vi "MFLI_Messgerät.vi"(1 "refnum":refnum<file>, 2 "Numerisch":i8 min=0 max=2 step=1) -> ()   [LabVIEW 2019]
uses:
  Global/Global Variables/Data_Display_global.vi
  Instrument_Setup.vi
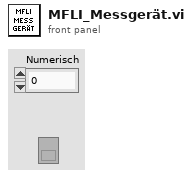
[diagram p1: front panel]
types:
  T1 = typedef "MFLIMonitor-Settings-Cluster.ctl" = cluster{"Adress":string, "Osc 0 Freq":dbl, "Osc 1 Freq":dbl, "Osc 2 Freq":dbl, "Osc 3 Freq":dbl, "Demod 0 Osc":i8, "Demod 0 Harm":i16, "Demod 0 Phase":dbl, "Demod 1 Osc":i8, "Demod 2 Osc":i8, "Demod 3 Osc":i8, "Demod 1 Harm":i16, "Demod 2 Harm":i16, "Demod 3 Harm":i16, "Demod 1 Phase":dbl, "Demod 2 Phase":dbl, "Demod 3 Phase":dbl, "Input Demod 0":string, "Input Demod 1":string, "Input Demod 2":string, "Input Demod 3":string, "Demod 0 Order":i8, "Demod 0 TC":dbl, "Demod 0 Sinc":bool, "Demod 1 Order":i8, "Demod 2 Order":i8, "Demod 3 Order":i8, "Demod 1 TC":dbl, "Demod 2 TC":dbl, "Demod 3 TC":dbl, "Demod 1 Sinc":bool, "Demod 2 Sinc":bool, "Demod 3 Sinc":bool, "Demod 0 Enable":bool, "Demod 0 Data Rate":dbl, "Demod 1 Enable":bool, "Demod 2 Enable":bool, "Demod 3 Enable":bool, "Demod 1 Data Rate":dbl, "Demod 2 Data Rate":dbl, "Demod 3 Data Rate":dbl, "Ampl 0":dbl, "Ampl 0 Enable":bool, "Ampl 1":dbl, "Ampl 2":dbl, "Ampl 3":dbl, "Ampl 1 Enable":bool, "Ampl 2 Enable":bool, "Ampl 3 Enable":bool, "On":bool, "50 Ohm":bool, "Range (V)":dbl, "Add":bool, "Diff":bool, "Auto-Range":bool, "Offset (V)":dbl, "Aux Out 0 Select":string, "Aux Out 0 Demod Num":dbl, "Aux Out 0 Pre Offset":dbl, "Aux Out 0 Scale":dbl, "Aux Out 0 Offset":dbl, "Aux Out 1 Select":string, "Aux Out 2 Select":string, "Aux Out 3 Select":string, "Aux Out 1 Pre Offset":dbl, "Aux Out 2 Pre Offset":dbl, "Aux Out 3 Pre Offset":dbl, "Aux Out 1 Scale":dbl, "Aux Out 2 Scale":dbl, "Aux Out 3 Scale":dbl, "Aux Out 1 Offset":dbl, "Aux Out 2 Offset":dbl, "Aux Out 3 Offset":dbl, "Aux Out 1 Demod Num":dbl, "Aux Out 2 Demod Num ":dbl, "Aux Out 3 Demod Num":dbl, "Output Range (V)":dbl}
  T2 = typedef "MFLIMonitor_Cluster.ctl" = cluster{"Demod 0":dbl[][], " Demod 1":dbl[][], "Demod 0 :X":dbl, "Demod 0 :Y ":dbl, "Demod 1 :X":dbl, "Demod 1 :Y ":dbl, " Demod 2":dbl[][], "Demod 3":dbl[][], "Demod 2 :X":dbl, "Demod 2 :Y ":dbl, "Demod 3 :X ":dbl, "Demod 3 :Y ":dbl, "Demod Sample out 0 ":T3, "Demod Sample out 1":T3, "Demod Sample out 2":T3, "Demod Sample out 3":T3, "Update Lock-In":bool, "Connected ?":bool, "Demod 0 Zero Phase":bool, "Demod 1 Zero Phase":bool, "Demod 2 Zero Phase":bool, "Demod 3 Zero Phase":bool, "Osc 0 Freq":dbl, "Osc 1 Freq":dbl, "Osc 2 Freq":dbl, "Osc 3 Freq":dbl, "Clipping":bool, "Range (V)":dbl, "Offset (V)":dbl, "Auto-Range":bool, "Add":bool, "Diff":bool, "On":bool, "50 Ohm":bool, "Ampl 0 Enable":bool, "Ampl 1 Enable":bool, "Ampl 2 Enable":bool, "Ampl 3 Enable":bool, "Ampl 0":dbl, "Ampl 1":dbl, "Ampl 2":dbl, "Ampl 3":dbl, "Update Osci":bool, "Output Range (V) ":dbl, "Set Range (in)":bool}
  T3 = typedef "Zurich Instruments LabOne.lvlib/ziTypeDemodSampleEx.ctl" = cluster{"Timestamps (ticks)":u64[], "X (Vrms)":dbl[], "Y (Vrms)":dbl[], "Osc Phase (rad)":dbl[], "Freq (Hz)":dbl[], "DIO":u32[], "Aux In 0 (V)":dbl[], "Aux In 1 (V)":dbl[], "Trigger":u32[]}
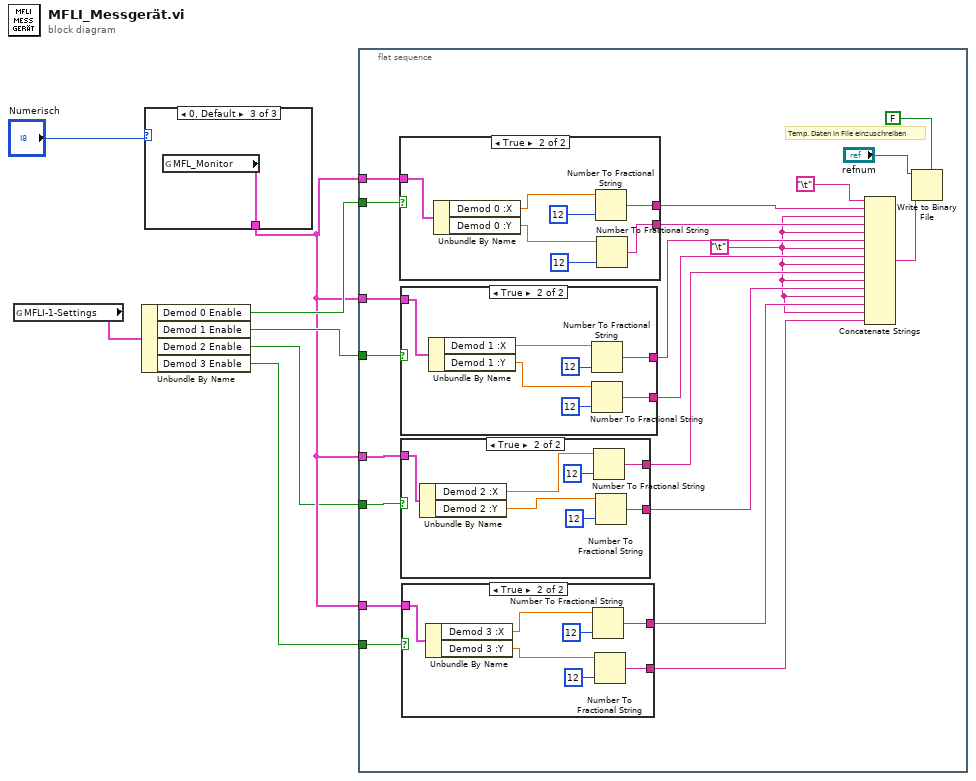
[diagram p0: block diagram]
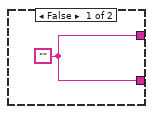
[diagram p2: hidden frame]
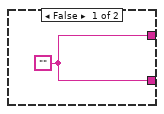
[diagram p3: hidden frame]
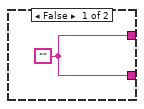
[diagram p4: hidden frame]
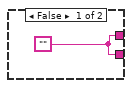
[diagram p5: hidden frame]
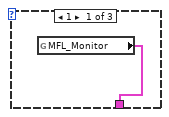
[diagram p6: hidden frame]
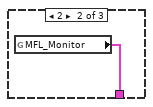
[diagram p7: hidden frame]
diagram:
  n1 = global read "Instrument_Setup.vi" "MFLI-1-Settings"() -> (w6:T1)
  n2 = Unbundle By Name(w6) -> ("Demod 0 Enable"=w5:bool, "Demod 1 Enable"=w4:bool, "Demod 2 Enable"=w2:bool, "Demod 3 Enable"=w1:bool)
  n3 = case shown="0, Default" "Numerisch" {
    tunnel: [w8 w9 w10] -> w3
    frame 1 {
      n4 = global read "Data_Display_global.vi" "MFL_Monitor"() -> (w8:T2)
    }
    frame 2 {
      n5 = global read "Data_Display_global.vi" "MFL_Monitor"() -> (w9:T2)
    }
    frame 0, Default {
      n6 = global read "Data_Display_global.vi" "MFL_Monitor"() -> (w10:T2)
    }
  }
  n7 = flat-sequence {
    tunnel: w3 -> [w21]
    tunnel: w5 -> [w20]
    tunnel: w4 -> [w19]
    tunnel: w3 -> [w18]
    tunnel: w3 -> [w17]
    tunnel: w3 -> [w16]
    tunnel: w2 -> [w15]
    tunnel: w1 -> [w14]
    frame #0 {
      w12 = "\t"
      # "Temp. Daten in File einzuschreiben"
      n8 = case shown="True" w20 {
        tunnel: [w56 w63] -> w29
        tunnel: [w56 w62] -> w28
        tunnel: w21 -> [_ w59]
        frame False {
          w56 = ""
        }
        frame True {
          n9 = Unbundle By Name(w59) -> ("Demod 0 :X"=w58:dbl, "Demod 0 :Y"=w57:dbl)
          n10 = Number To Fractional String(number=w58, precision (6)=i16 12) -> (F-format string=w63:string)  [unwired: 2 in]
          n11 = Number To Fractional String(number=w57, precision (6)=i16 12) -> (F-format string=w62:string)  [unwired: 2 in]
        }
      }
      n12 = case shown="True" w19 {
        tunnel: [w48 w55] -> w25
        tunnel: [w48 w52] -> w24
        tunnel: w18 -> [_ w51]
        frame False {
          w48 = ""
        }
        frame True {
          n13 = Unbundle By Name(w51) -> ("Demod 1 :X"=w50:dbl, "Demod 1 :Y"=w49:dbl)
          n14 = Number To Fractional String(number=w50, precision (6)=i16 12) -> (F-format string=w55:string)  [unwired: 2 in]
          n15 = Number To Fractional String(number=w49, precision (6)=i16 12) -> (F-format string=w52:string)  [unwired: 2 in]
        }
      }
      n16 = case shown="True" w15 {
        tunnel: [w40 w45] -> w23
        tunnel: [w40 w44] -> w22
        tunnel: w17 -> [_ w43]
        frame False {
          w40 = ""
        }
        frame True {
          n17 = Unbundle By Name(w43) -> ("Demod 2 :X"=w42:dbl, "Demod 2 :Y"=w41:dbl)
          n18 = Number To Fractional String(number=w42, precision (6)=i16 12) -> (F-format string=w45:string)  [unwired: 2 in]
          n19 = Number To Fractional String(number=w41, precision (6)=i16 12) -> (F-format string=w44:string)  [unwired: 2 in]
        }
      }
      n20 = case shown="True" w14 {
        tunnel: w16 -> [_ w37]
        tunnel: [w32 w34] -> w13
        tunnel: [w32 w33] -> w11
        frame False {
          w32 = ""
        }
        frame True {
          n21 = Unbundle By Name(w37) -> ("Demod 3 :X"=w36:dbl, "Demod 3 :Y"=w35:dbl)
          n22 = Number To Fractional String(number=w36, precision (6)=i16 12) -> (F-format string=w34:string)  [unwired: 2 in]
          n23 = Number To Fractional String(number=w35, precision (6)=i16 12) -> (F-format string=w33:string)  [unwired: 2 in]
        }
      }
      n24 = Concatenate Strings("\t", w29, w12, w28, w12, w25, w12, w24, w12, w23, w12, w22, w12, w13, w12, w11) -> (w31:string)
      n25 = Write to Binary File ("Write File")(file (use dialog)="refnum", data=w31, 5:FALSE ("prepend array or string size? (T)")) -> ()  [unwired: 3 in, 3 out]
    }
  }
